vi "Open_file_set_refnum.vi"(8 "error in (no error)":errorcluster, 11 "HIS in":refnum<class "HIS.lvclass">) -> (0 "error out":errorcluster, 3 "HIS out":refnum<class "HIS.lvclass">)   [LabVIEW 2015, in "HIS.lvclass"]
uses:
  HIS.lvclass
  DATA.lvclass
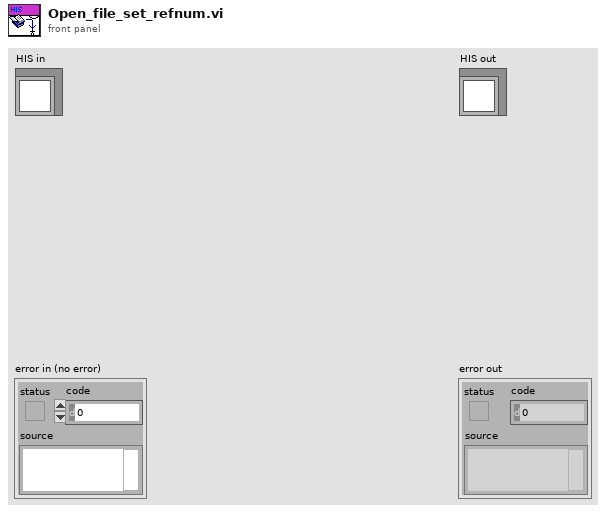
[diagram p1: front panel]
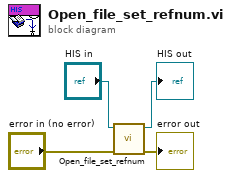
[diagram p0: block diagram]
diagram:
  n1 = call-parent "Open_file_set_refnum.vi"("error in (no error)"="error in (no error)", "DATA in"="HIS in") -> ("error out"=→"error out":errorcluster, "DATA out"=→"HIS out":refnum<class "HIS.lvclass">)  [unwired: 8 in]
